vi "Find cDAQ.vi"() -> ()   [LabVIEW 2019]
uses:
  <vilib>/nisyscfg/nisyscfg.lvlib
  <vilib>/nisyscfg/Filter Mode.ctl
  <resource>/objmgr/nisysapi.rc
  <resource>/objmgr/nicontrollersysapi.rc
  Type Defs and Controls/System Type.ctl
  Type Defs and Controls/Registered System.ctl
  <vilib>/DAQmx/read.llb/DAQmx Read (Analog 2D DBL NChan NSamp).vi
panel:
  out "data":dbl[][](array[numeric]) format="%0.2f"
  out "error out":errorcluster
  out "Devices & Chassis:Bus Specific:TCP/IP Hostname":string
  out "Devices & Chassis:Product Name":string
  out "Detected Systems":string[](array[string])
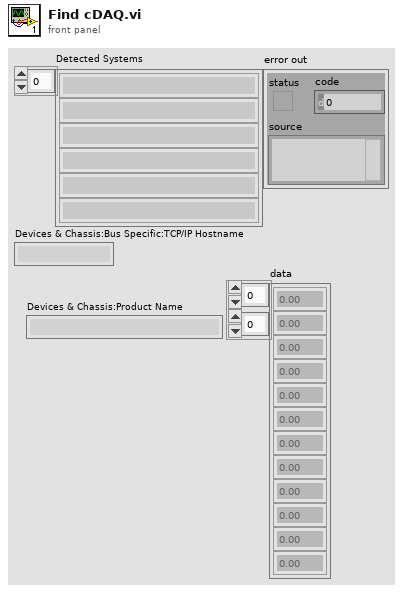
[diagram p1: front panel]
types:
  T1 = typedef "Registered System.ctl" = cluster{"System Type":T2, "Serial Number":u32, "ID":string, "Cal File?":bool}
  T2 = typedef "System Type.ctl" = enum16{"DAQ Rack", "DAQ Cart", "nx-5000", "unknown", "open"}
  T3 = typedef "nisyscfg.lvlib/Filter Mode.ctl" = i32
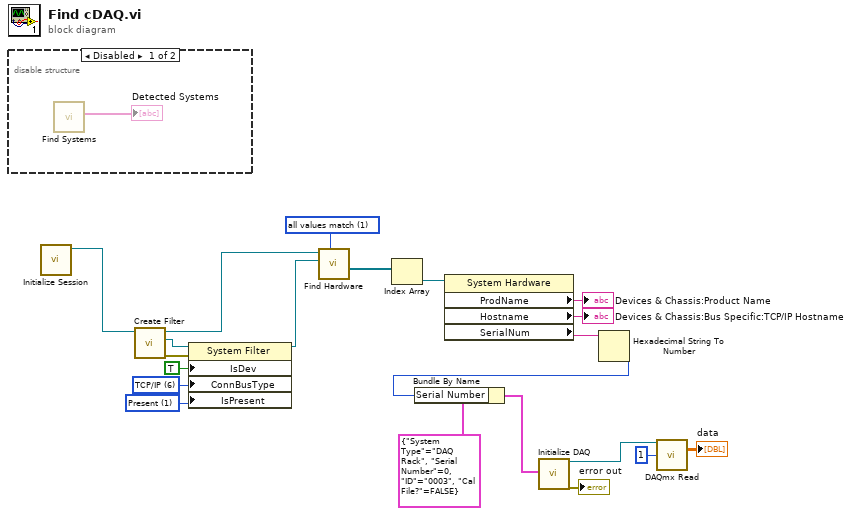
[diagram p0: block diagram]
diagram:
  w1 = 1 items=["Initializing"=-2, "Unknown"=-1, "Not Present"=0, "Present"=1] ("Devices & Chassis:Is Present")
  w14 = u32 6 items=["BuiltIn/System", "PXI/PCI", "USB", "GPIB", "VXI", "Serial", "TCP/IP", "cRIO", "SCXI", "cDAQ", "SwitchBlock", "SCC", "FireWire", "Accessory", "CAN", "SwitchBlock Device"] ("Devices & Chassis:Connects To Bus Type")
  w21 = T3 1 items=["all values match"=1, "any value matches"=2, "values do not match"=3, "all properties exist"=4] ("Filter Mode (all values match)")
  n1 = disable-structure shown="Disabled" {
    frame Disabled {
      n2 = call <vilib>:"Find Systems.vi"() -> ("Detected Systems"=→"Detected Systems":string[])  [unwired: 9 in, 2 out]
    }
    frame Enabled {
    }
  }
  n3 = call <vilib>:"Initialize Session.vi"() -> ("Session out"=w17:refnum<k21>)  [unwired: 10 in, 1 out]
  n4 = call <vilib>:"Create Filter.vi"("Session in"=w17) -> ("error out"=w20:errorcluster, "Filter out"=w19:refnum<k20>, "Session out"=w16:refnum<k21>)  [unwired: 8 in]
  n5 = property class="System Filter"(reference=w19, error in=w20, "IsDev"=TRUE ("Is Chassis"), "ConnBusType"=w14, "IsPresent"=w1) -> (reference out=w15:refnum<k20>)  [unwired: 1 out]
  n6 = call <vilib>:"Find Hardware.vi"("Filter Mode (all values match)"=w21, "Filter in"=w15, "Session in"=w16) -> ("Resources out"=w13:refnum<k20>[])  [unwired: 5 in, 3 out]
  n7 = Index Array(array=w13) -> (element=w12:refnum<k20>)  [unwired: 1 in]
  n8 = property class="System Hardware"(reference=w12) -> ("ProdName"=→"Devices & Chassis:Product Name":string, "Hostname"=→"Devices & Chassis:Bus Specific:TCP/IP Hostname":string, "SerialNum"=w7:string)  [unwired: 1 in, 2 out]
  n9 = Hexadecimal String To Number(string=w7) -> (number=w6:u32)  [unwired: 2 in, 1 out]
  n10 = Bundle By Name(cluster=T1 {"System Type"=enum."DAQ Rack", "Serial Number"=0, "ID"="0003", "Cal File?"=FALSE} ("System"), "Serial Number"=w6) -> (w8:T1)
  n11 = call "Initialize DAQ.vi"(2:w8) -> ("AI Task OUT"=w4:refnum<k21>, "error out"=→"error out":errorcluster)  [unwired: 17 in]
  n12 = call-poly <vilib>:"DAQmx Read.vi"("task/channels in"=w4, "number of samples per channel"=1) -> ("data"=→"data":dbl[][])  [unwired: 11 in, 2 out]
